vi "PCI Configuration.Get Register Offset.vi"(11 "PCI Configuration Register":T1) -> (3 "Offset":u32)   [LabVIEW 2016, in "GE 5565PIORC.lvclass"]
uses:
  GE 5565PIORC.lvclass
  Controls/Registers.PCI Configuration.ctl
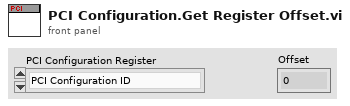
[diagram p1: front panel]
types:
  T1 = typedef "GE 5565PIORC.lvclass/Registers.PCI Configuration.ctl" = enum16{"PCI Configuration ID", "PCI Command", "PCI Status", "PCI Revision ID", "PCI Class Code", "PCI Cache Line Size", "PCI Latency Timer", "PCI Header Type", "PCI Built-In Self-Test", "PCI BAR 0", "PCI BAR 1", "PCI BAR 2", "PCI BAR 3", "PCI BAR 4", "PCI BAR 5", "PCI Cardbus CIS Pointer", "PCI Subsystem Vendor ID", "PCI Subsytem ID", "PCI Expansion ROM Base", "PCI Capability Pointer", "PCI Interrupt Line", "PCI Interrupt Pin", "PCI Min_Gnt", "PCI Max_Lat"}
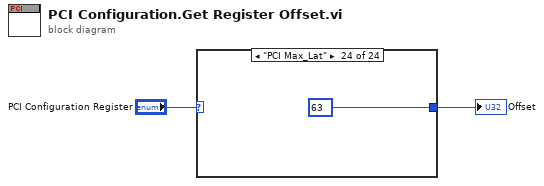
[diagram p0: block diagram]
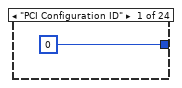
[diagram p2: hidden frame]
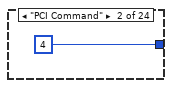
[diagram p3: hidden frame]
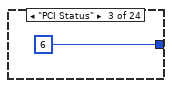
[diagram p4: hidden frame]
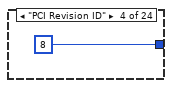
[diagram p5: hidden frame]
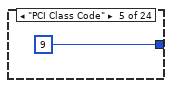
[diagram p6: hidden frame]
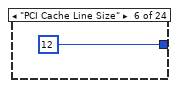
[diagram p7: hidden frame]
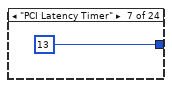
[diagram p8: hidden frame]
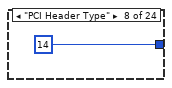
[diagram p9: hidden frame]
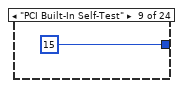
[diagram p10: hidden frame]
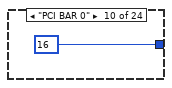
[diagram p11: hidden frame]
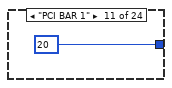
[diagram p12: hidden frame]
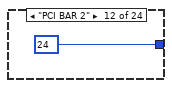
[diagram p13: hidden frame]
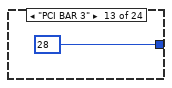
[diagram p14: hidden frame]
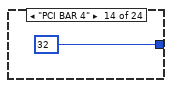
[diagram p15: hidden frame]
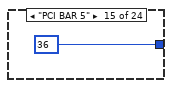
[diagram p16: hidden frame]
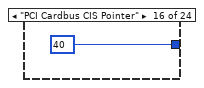
[diagram p17: hidden frame]
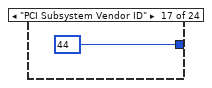
[diagram p18: hidden frame]
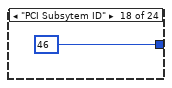
[diagram p19: hidden frame]
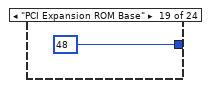
[diagram p20: hidden frame]
diagram:
  n1 = case shown="\"PCI Max_Lat\"" "PCI Configuration Register" {
    tunnel: [u32 0 u32 4 u32 6 u32 8 u32 9 u32 12 u32 13 u32 14 u32 15 u32 16 u32 20 u32 24 u32 28 u32 32 u32 36 u32 40 u32 44 u32 46 u32 48 u32 52 u32 60 u32 61 u32 62 u32 63] -> w2
    frame "PCI Configuration ID" {
    }
    frame "PCI Command" {
    }
    frame "PCI Status" {
    }
    frame "PCI Revision ID" {
    }
    frame "PCI Class Code" {
    }
    frame "PCI Cache Line Size" {
    }
    frame "PCI Latency Timer" {
    }
    frame "PCI Header Type" {
    }
    frame "PCI Built-In Self-Test" {
    }
    frame "PCI BAR 0" {
    }
    frame "PCI BAR 1" {
    }
    frame "PCI BAR 2" {
    }
    frame "PCI BAR 3" {
    }
    frame "PCI BAR 4" {
    }
    frame "PCI BAR 5" {
    }
    frame "PCI Cardbus CIS Pointer" {
    }
    frame "PCI Subsystem Vendor ID" {
    }
    frame "PCI Subsytem ID" {
    }
    frame "PCI Expansion ROM Base" {
    }
    frame "PCI Capability Pointer" {
    }
    frame "PCI Interrupt Line" {
    }
    frame "PCI Interrupt Pin" {
    }
    frame "PCI Min_Gnt" {
    }
    frame "PCI Max_Lat" {
    }
  }
  "Offset" <- w2
